vi "(SubVI) Odijk eWLC fitting.vi"(4 "Force (pN)":dbl[](array[numeric]), 5 "Extension (nm)":dbl[](array[numeric]), 7 "initial parameters for eWLC (Lp,Lc,K=1200)":dbl[](array[numeric])=[45.0, 1500.0, 1200.0]) -> (0 "Force to fit":dbl[](array[numeric]), 1 "r^2":dbl, 2 "best nonlinear fit for Extension (nm)":dbl[](array[numeric]), 3 "best fit parameters\n(Lp,Lc,K=1200)":dbl[](array[numeric]))   [LabVIEW 2014]
uses:
  <vilib>/gmath/NumericalOptimization/Nonlinear Curve Fit LM formula string.vi
  <vilib>/gmath/NI_Gmath.lvlib
panel:
  out "residue":dbl
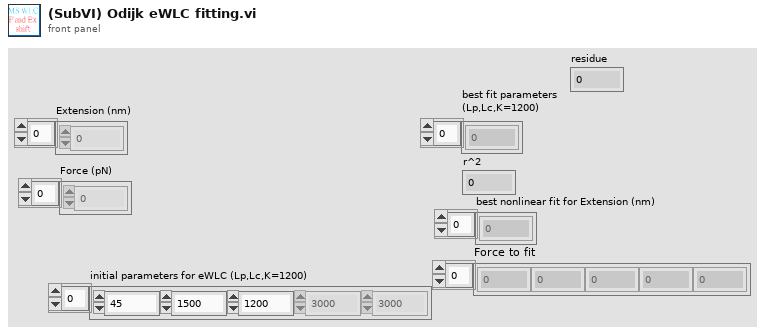
[diagram p1: front panel]
types:
  T1 = cluster{"model":string, "Parameters":string[], "x":string}
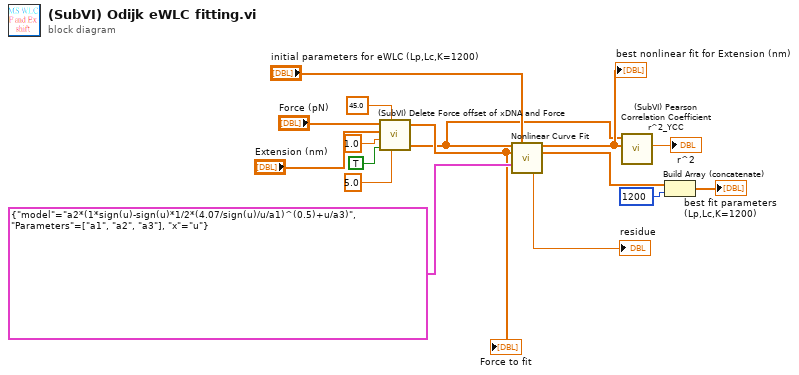
[diagram p0: block diagram]
diagram:
  n1 = call "(SubVI) Delete Force offset of xDNA and Force.vi"("Force"="Force (pN)", "Upper Force (pN)"=45.0, "xDNA"="Extension (nm)", "force constant"=1.0, "Lower Force (pN)"=5.0, "Set lower foce offset?"=TRUE) -> ("cut-full Force"=w5:dbl[], "cut-full xDNA"=w4:dbl[])  [unwired: 1 in]
  "Force to fit" <- w5
  n2 = call-poly <vilib>:"Nonlinear Curve Fit.vi"("Y"=w4, "initial parameters"="initial parameters for eWLC (Lp,Lc,K=1200)", "X"=w5, "model description"=T1 {"model"="a2*(1*sign(u)-sign(u)*1/2*(4.07/sign(u)/u/a1)^(0.5)+u/a3)", "Parameters"=["a1", "a2", "a3"], "x"="u"}) -> ("best nonlinear fit"=w14:dbl[], "best fit parameters"=w3:dbl[], "residue"=→"residue":dbl)  [unwired: 3 in, 6 out]
  "best nonlinear fit for Extension (nm)" <- w14
  n3 = call "(SubVI) Pearson Correlation Coefficient r^2_YCC.vi"("best fit Data"=w14, "Data"=w4) -> ("r^2"=→"r^2":dbl)  [unwired: 4 in, 1 out]
  n4 = Build Array (concatenate)(w3, 1200 ("Numeric")) -> (→"best fit parameters\n(Lp,Lc,K=1200)":dbl[])
